vi "insert values.vi"(4 "数据库类型":T2, 5 "是否创建唯一键":bool, 7 "data":variant[](array[variant]), 8 "错误输入（无错误）":errorcluster, 9 "columns外部输入":T1, 10 "database":string="database1", 11 "Tabe Name":string) -> (0 "错误输出":errorcluster)   [LabVIEW 2016]
uses:
  Access/Access Lib.lvlib
  SQLite/SQLite Lib.lvlib
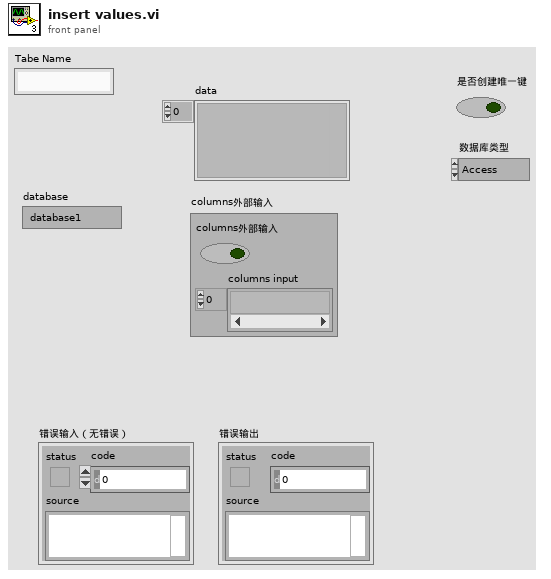
[diagram p1: front panel]
types:
  T1 = cluster{"columns外部输入":bool, "columns input":string[]}
  T2 = typedef "数据库类型.ctl" = enum16{"Access", "SQLite"}
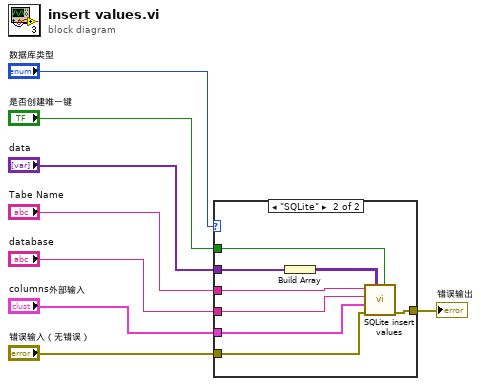
[diagram p0: block diagram]
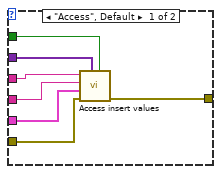
[diagram p2: hidden frame]
diagram:
  n1 = case shown="\"SQLite\"" "数据库类型" {
    tunnel: "Tabe Name" -> [w11 w23]
    tunnel: "是否创建唯一键" -> [w14 w22]
    tunnel: "错误输入（无错误）" -> [w13 w21]
    tunnel: [w12 w20] -> w5
    tunnel: "data" -> [w15 w19]
    tunnel: "database" -> [w10 w17]
    tunnel: "columns外部输入" -> [w9 w16]
    frame "Access", Default {
      n2 = call "Access insert values.vi"("是否创建唯一键"=w14, "data"=w15, "error in (no error)"=w13, "columns外部输入"=w9, "database"=w10, "table"=w11) -> ("error out"=w12:errorcluster)  [unwired: 5 in]
    }
    frame "SQLite" {
      n3 = Build Array(w19) -> (w18:variant[][])
      n4 = call "SQLite insert values.vi"("是否创建唯一键"=w22, "数组"=w18, "错误输入（无错误）"=w21, "columns外部输入"=w16, "database"=w17, "Tabe Name"=w23) -> ("错误输出"=w20:errorcluster)  [unwired: 5 in]
    }
  }
  "错误输出" <- w5
